vi "array_angles.vi"(11 "Array":i32[][](array[numeric])) -> (3 "Array 2":i32[][](array[numeric]))   [LabVIEW 2014]
panel:
  out "XY Graph":cluster{"Y":dbl[], "Y":dbl[]}[](graph)
  out "Array 5":dbl[][](array[numeric])
  out "Array 4":dbl[][](array[numeric])
  out "Array 3":i32[][](array[numeric])
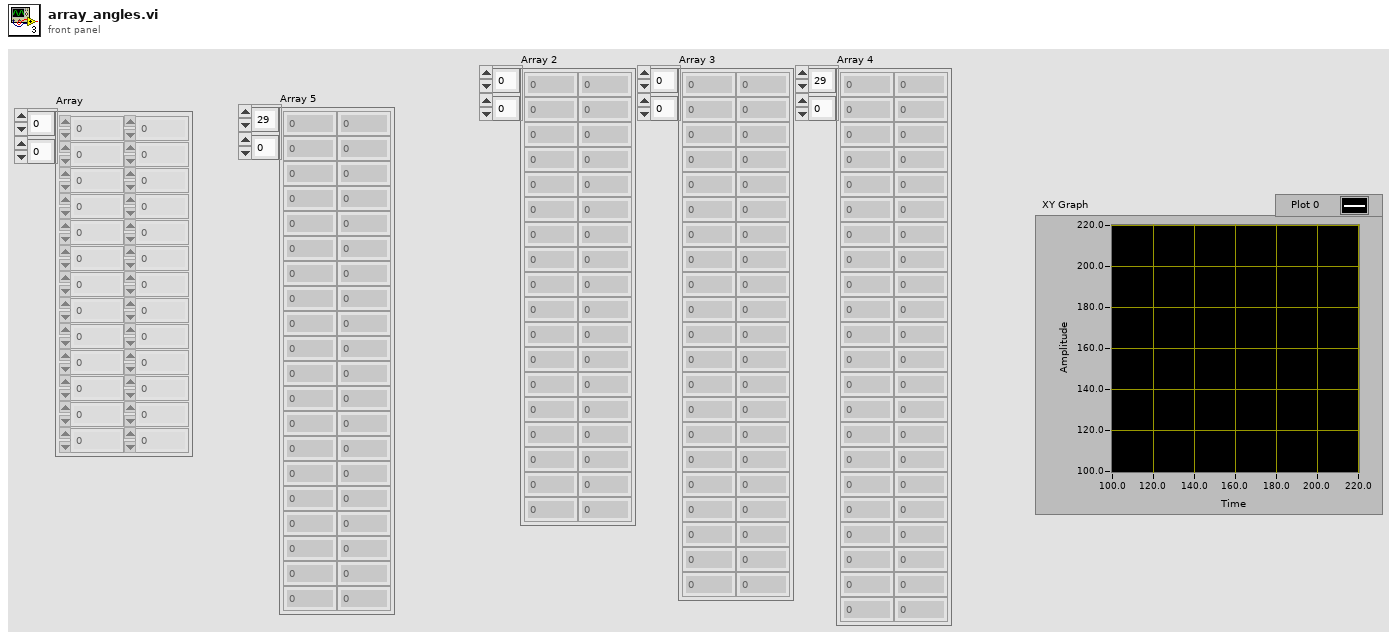
[diagram p1: front panel]
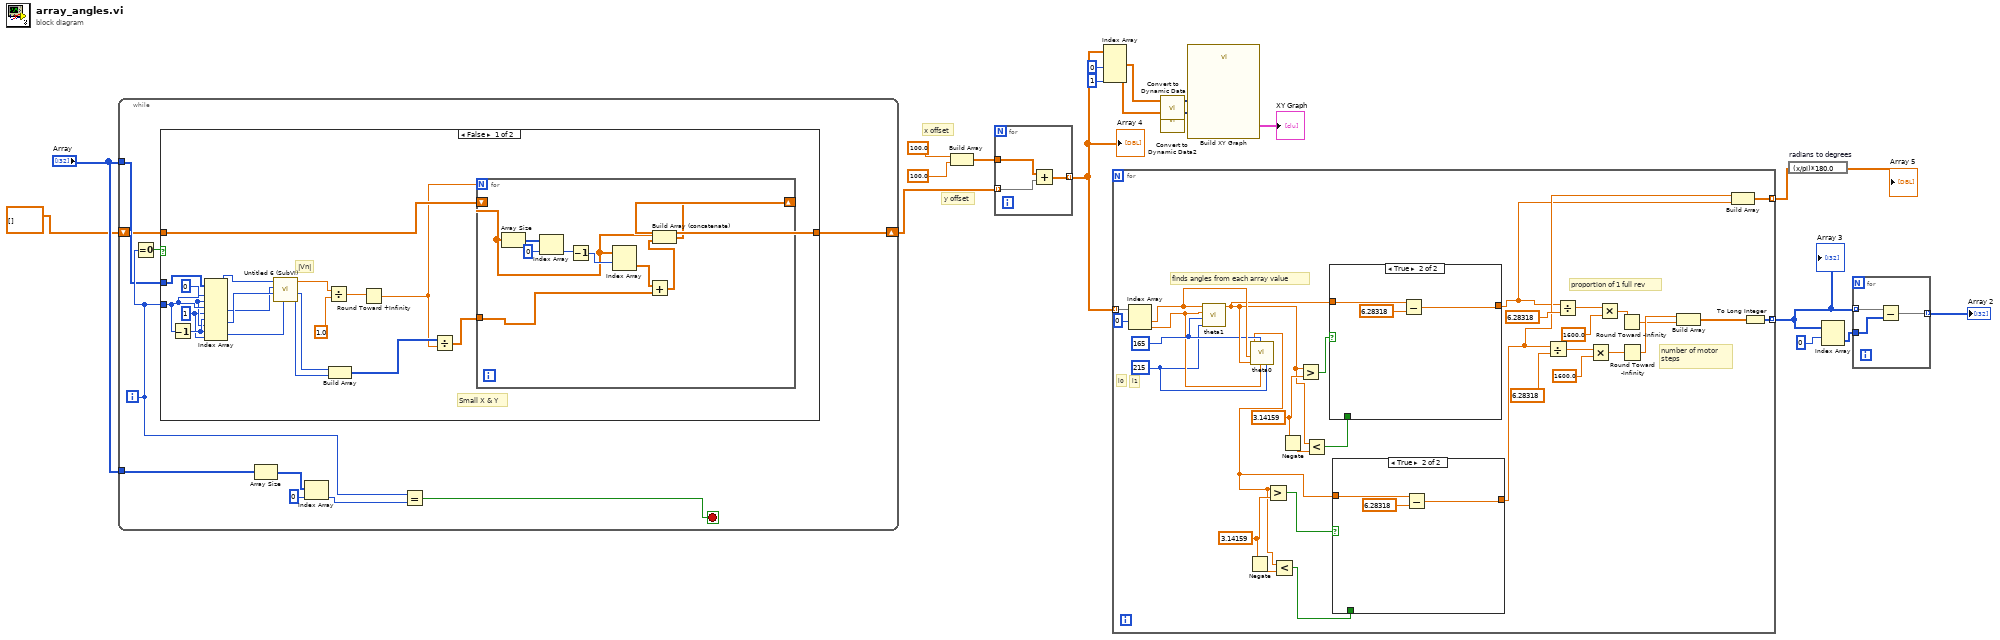
[diagram p0: block diagram]
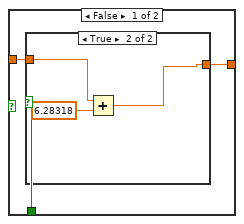
[diagram p2: hidden frame]
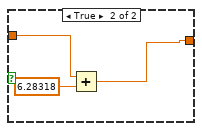
[diagram p5: hidden frame]
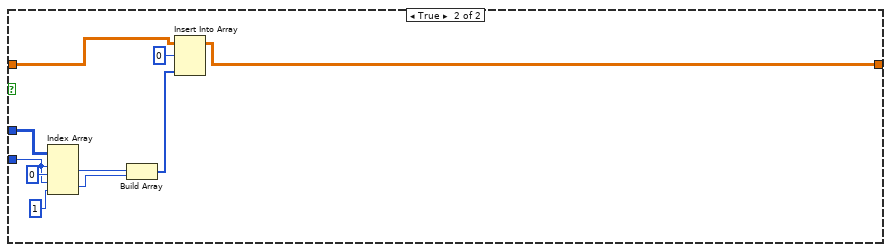
[diagram p6: hidden frame]
diagram:
  # "y offset"
  # "x offset"
  n1 = while {
    tunnel: "Array" -> [w23]
    tunnel: "Array" -> [w30]
    shift-right: [w21] -> w16
    shift-left: dbl[][] [] -> [w22]
    i -> [w24]
    stop <- w26 stop-if-true
    n2 = Equal To 0?(x=w24) -> (x = 0?=w25:bool)
    n3 = case shown="False" w25 {
      tunnel: w24 -> [w48 w65]
      tunnel: w23 -> [w49 w66]
      tunnel: w22 -> [w44 w64]
      tunnel: [w43 w59] -> w21
      frame False {
        w45 = 1 ("disabled index (col)")
        w46 = 0 ("disabled index (col)")
        # "|Vn|"
        # "Small X & Y"
        n4 = Decrement(x=w48) -> (x-1=w47:i32)
        n5 = Index Array(array=w49, index (row) #1=w48, index (col) #1=w46, index (row) #2=w48, index (col) #2=w45, index (row) #3=w47, index (col) #3=w46, index (row) #4=w47, index (col) #4=w45) -> (element #1=w42:i32, element #2=w40:i32, element #3=w41:i32, element #4=w39:i32)
        n6 = call "Untitled 6 (SubVI).vi"("Numeric in"=w39, "Numeric 4"=w41, "Numeric 3"=w40, "Numeric 5"=w42) -> ("y"=w34:i32, "x"=w35:i32, "Numeric out"=w38:dbl)  [unwired: 5 in]
        n7 = Divide(x=w38, y=1.0) -> (x/y=w36:dbl)
        n8 = Build Array(w35, w34) -> (w33:i32[])
        n9 = Round Toward +Infinity(x=w36) -> (ceil(x): smallest int >= x=w31:dbl)
        n10 = Divide(x=w33, y=w31) -> (x/y=w32:dbl[])
        n11 = for {
          N: w31 -> [_]
          tunnel: w32 -> [w53]
          shift-right: [w51] -> w43
          shift-left: w44 -> [w50]
          n12 = Array Size(array=w50) -> (size(s)=w58:i32[])
          n13 = Index Array(array=w58, index=0) -> (element=w56:i32)
          n14 = Decrement(x=w56) -> (x-1=w55:i32)
          n15 = Index Array(array=w50, index (row)=w55) -> (element=w54:dbl[])  [unwired: 1 in]
          n16 = Add(x=w54, y=w53) -> (x+y=w52:dbl[])
          n17 = Build Array (concatenate)(w50, w52) -> (w51:dbl[][])
        }
      }
      frame True {
        n18 = Index Array(array=w66, index (row) #1=w65, index (col) #1=0 ("disabled index (col)"), index (row) #2=w65, index (col) #2=1 ("disabled index (col)")) -> (element #1=w62:i32, element #2=w61:i32)
        n19 = Build Array(w62, w61) -> (w60:i32[])
        n20 = Insert Into Array(array=w64, index (row)=0, new element=w60) -> (w59:dbl[][])  [unwired: 1 in]
      }
    }
    n21 = Array Size(array=w30) -> (size(s)=w29:i32[])
    n22 = Index Array(array=w29, index=0) -> (element=w27:i32)
    n23 = Equal?(x=w24, y=w27) -> (x = y?=w26:bool)
  }
  n24 = Build Array(100.0, 100.0) -> (w15:dbl[])
  n25 = for {
    tunnel: w16 -> [w71] mode=indexing
    tunnel: w15 -> [w70]
    tunnel: [w69] -> w7 mode=indexing
    n26 = Add(x=w70, y=w71) -> (x+y=w69:dbl[])
  }
  "Array 4" <- w7
  n27 = Index Array(array=w7, index (col) #1=0 ("disabled index (col)"), index (col) #2=1 ("index (col)")) -> (element #1=w4:dbl[], element #2=w2:dbl[])  [unwired: 2 in]
  n28 = for {
    tunnel: w7 -> [w102] mode=indexing
    tunnel: [w85] -> w12 mode=indexing
    tunnel: [w81] -> w10 mode=indexing
    w89 = 3.14159 ("y")
    w92 = 3.14159 ("y")
    w73 = 215 ("L0")
    w75 = 165 ("L0")
    # "number of motor\nsteps"
    # "proportion of 1 full rev"
    # "finds angles from each array value"
    # "l1"
    # "l0"
    n29 = Index Array(array=w102, index #1=0 ("index")) -> (element #1=w77:dbl, element #2=w74:dbl)  [unwired: 1 in]
    n30 = call "theta1.vi"("L1"=w73, "l0"=w75, "Numeric 2"=w74, "Numeric"=w77) -> ("Numeric 5"=w76:dbl)  [unwired: 7 in]
    n31 = Negate(x=w89) -> (-x=w88:dbl)
    n32 = call "theta0.vi"("L1"=w73, "X"=w74, "L0"=w75, "theta 1"=w76, "Y"=w77) -> ("theta 0"=w72:dbl)  [unwired: 6 in]
    n33 = Greater?(x=w72, y=w89) -> (0:w87:bool)
    n34 = Less?(x=w72, y=w88) -> (x < y?=w86:bool)
    n35 = Negate(x=w92) -> (-x=w91:dbl)
    n36 = Greater?(x=w76, y=w92) -> (0:w93:bool)
    n37 = Less?(x=w76, y=w91) -> (x < y?=w90:bool)
    n38 = case shown="True" w93 {
      tunnel: w76 -> [w113 w122]
      tunnel: w90 -> [w115 _]
      tunnel: [w114 w120] -> w78
      frame False {
        n39 = case shown="False" w115 {
          tunnel: [w116 w117] -> w114
          tunnel: w113 -> [w116 w118]
          frame False {
          }
          frame True {
            n40 = Add(x=w118, y=6.28318) -> (x+y=w117:dbl)
          }
        }
      }
      frame True {
        n41 = Subtract(x=w122, y=6.28318) -> (x-y=w120:dbl)
      }
    }
    n42 = case shown="True" w87 {
      tunnel: w72 -> [w103 w112]
      tunnel: w86 -> [w105 _]
      tunnel: [w104 w110] -> w79
      frame False {
        n43 = case shown="True" w105 {
          tunnel: [w106 w107] -> w104
          tunnel: w103 -> [w106 w108]
          frame False {
          }
          frame True {
            n44 = Add(x=w108, y=6.28318) -> (x+y=w107:dbl)
          }
        }
      }
      frame True {
        n45 = Subtract(x=w112, y=6.28318) -> (x-y=w110:dbl)
      }
    }
    n46 = Divide(x=w79, y=6.28318) -> (x/y=w96:dbl)
    n47 = Divide(x=w78, y=6.28318) -> (x/y=w100:dbl)
    n48 = Multiply(x=w96, y=1600.0) -> (x*y=w94:dbl)
    n49 = Multiply(x=w100, y=1600.0) -> (x*y=w98:dbl)
    n50 = Round Toward -Infinity(1:w98) -> (0:w82:dbl)
    n51 = Round Toward -Infinity(1:w94) -> (0:w83:dbl)
    n52 = Build Array(w83, w82) -> (w84:dbl[])
    n53 = Build Array(w79, w78) -> (w81:dbl[])
    n54 = To Long Integer(number=w84) -> (32bit integer=w85:i32[])
  }
  "Array 3" <- w12
  n55 = call "Convert to Dynamic Data"("Array"=w4) -> ("Dynamic Data Type"=w3:dynamicdata)  [unwired: 3 in]
  n56 = call "Convert to Dynamic Data2"("Array"=w2) -> ("Dynamic Data Type"=w1:dynamicdata)  [unwired: 3 in]
  n57 = call "Build XY Graph"("Y Input"=w1, "X Input"=w3) -> ("XY Graph"=→"XY Graph":cluster{"X":dbl[], "Y":dbl[]}[])  [unwired: 8 in, 1 out]
  n58 = expression code="(x/pi)*180.0" "radians to degrees"(w10) -> (→"Array 5":dbl[][])
  n59 = Index Array(array=w12, index (row)=0) -> (element=w13:i32[])  [unwired: 1 in]
  n60 = for {
    tunnel: w13 -> [w124]
    tunnel: w12 -> [w125] mode=indexing
    tunnel: [w123] -> w11 mode=indexing
    n61 = Subtract(x=w125, y=w124) -> (x-y=w123:i32[])
  }
  "Array 2" <- w11
